vi "Force sensor FPGA test.vi"(8 "FPGA I/O In 4":refnum<k21>="Connector0/AI0", 9 "FPGA I/O In 3":refnum<k21>="Connector0/AI0", 10 "FPGA I/O In 2":refnum<k21>="Connector0/AI0", 11 "FPGA I/O In":refnum<k21>="Connector0/AI0") -> (0 "I/O Item 4":i16, 1 "I/O Item 3":i16, 2 "I/O Item 2":i16, 3 "I/O Item":i16)   [LabVIEW 2018, in "jmslib.lvlib"]
uses:
  jmslib.lvlib
  <vilib>/rvi/eio/common/nirviEmuTemplateMethod_errors.vi
  <vilib>/eio/EIONode/EIONode.xnode
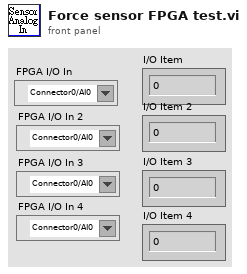
[diagram p1: front panel]
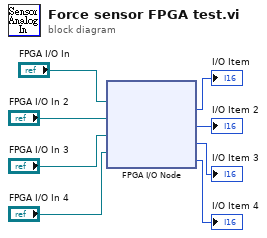
[diagram p0: block diagram]
diagram:
  n1 = xnode "FPGA I/O Node"("FPGA I/O In"="FPGA I/O In", "FPGA I/O In"="FPGA I/O In 2", "FPGA I/O In"="FPGA I/O In 3", "FPGA I/O In"="FPGA I/O In 4") -> ("I/O Item"=→"I/O Item":i16, "I/O Item"=→"I/O Item 2":i16, "I/O Item"=→"I/O Item 3":i16, "I/O Item"=→"I/O Item 4":i16)  [unwired: 4 out]
